vi "Array to File.vi"(8 "error in":errorcluster, 10 "array in":T1[](array[typedef]) {"Creation Date" format="%<%x>T"; "Last Updated" format="%<%x>T"}, 11 "file path in":path) -> (0 "error out":errorcluster, 3 "file path out":path)   [LabVIEW 2018]
uses:
  Type Defs/SR Cluster.ctl
  Type Defs/SR Status.ctl
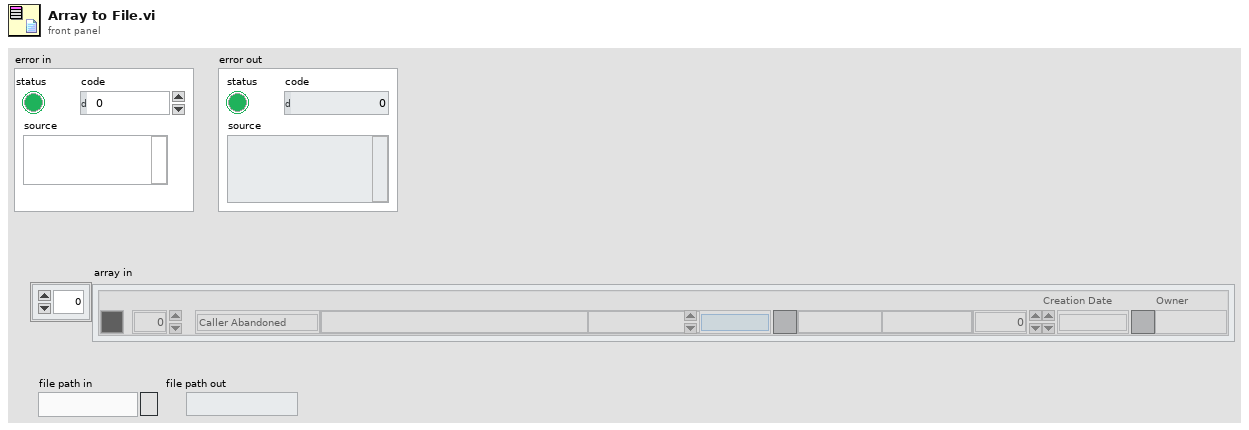
[diagram p1: front panel]
types:
  T1 = typedef "SR Cluster.ctl" = cluster{"Color":u32, "SR Number":i32, "SR Status":T2, "Name":string, "Summary":string, "Last Updated":timestamp, "SR Type":string, "Service Level":string, "Days Open":dbl, "Creation Date":timestamp, "Owner":string}
  T2 = typedef "SR Status.ctl" = enum16{"Caller Abandoned", "Created in Error", "Expired", "Forum Resolved AE", "Forum Resolved Customer", "IN WORK", "IN WORK Collab with AES", "IN WORK Collab with PSE", "IN WORK Collab with SE", "IN WORK Customer Added Note", "IN WORK Escalation", "IN WORK Wait on Customer", "Open", "Potentially Resolved", "Presumed Resolved", "RMA Approved for Return", "RMA Closed", "RMA Closed - DOA", "RMA In Progress", "RMA Open", "RMA Waiting on Customer", "Resolved", "Passed Off"}
  T3 = enum16{"open", "replace", "create", "open or create", "replace or create", "replace or create with confirmation"}
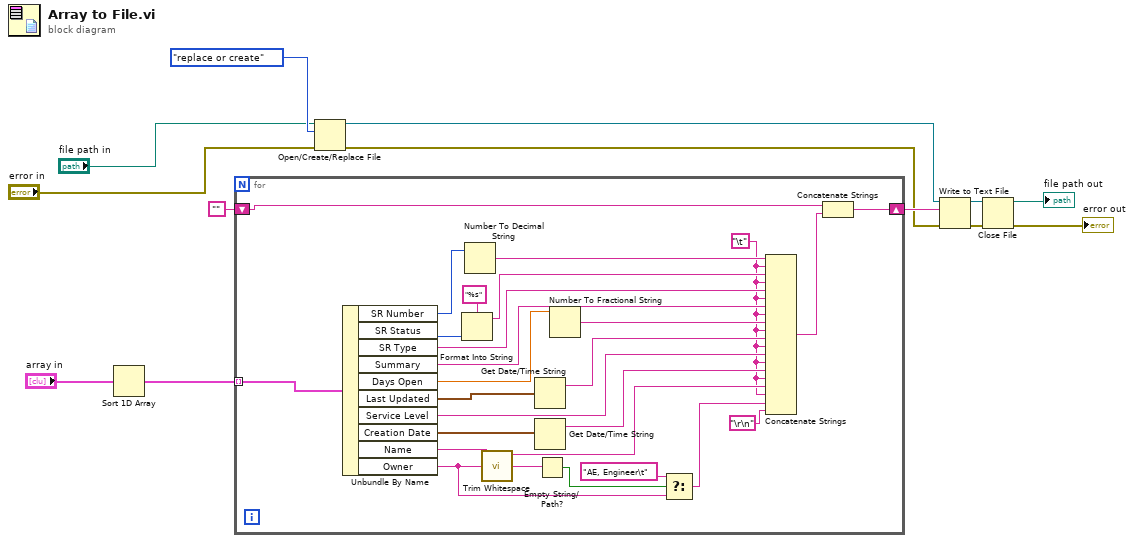
[diagram p0: block diagram]
diagram:
  n1 = Sort 1D Array(array="array in") -> (sorted array=w1:T1[])
  n2 = for {
    shift-right: [w39] -> w11
    shift-left: "" -> [w38]
    tunnel: w1 -> [w24] mode=indexing
    w15 = "\t"
    n3 = Unbundle By Name(w24) -> ("SR Number"=w36:i32, "SR Status"=w27:T2, "SR Type"=w34:string, "Summary"=w28:string, "Days Open"=w33:dbl, "Last Updated"=w29:timestamp, "Service Level"=w30:string, "Creation Date"=w23:timestamp, "Name"=w21:string, "Owner"=w17:string)
    n4 = Format Into String(format string="%s", w27) -> (resulting string=w25:string)  [unwired: 2 in, 1 out]
    n5 = Number To Decimal String(number=w36) -> (decimal integer string=w35:string)  [unwired: 1 in]
    n6 = call <vilib>:"Trim Whitespace.vi"("string"=w17) -> ("trimmed string"=w19:string)  [unwired: 1 in]
    n7 = Get Date/Time String(seconds (now)=w29) -> (date string=w31:string)  [unwired: 2 in, 1 out]
    n8 = Get Date/Time String(seconds (now)=w23) -> (date string=w22:string)  [unwired: 2 in, 1 out]
    n9 = Empty String/Path?(string/path=w19) -> (empty?=w18:bool)
    n10 = Number To Fractional String(number=w33) -> (F-format string=w32:string)  [unwired: 3 in]
    n11 = Select(t="AE, Engineer\t", s=w18, f=w17) -> (s? t:f=w14:string)
    n12 = Concatenate Strings(w35, w15, w25, w15, w34, w15, w28, w15, w32, w15, w31, w15, w30, w15, w22, w15, w21, w15, w14, "\r\n") -> (w37:string)
    n13 = Concatenate Strings(w38, w37) -> (w39:string)
  }
  n14 = Open/Create/Replace File(file path (use dialog)="file path in", error in="error in", operation (0:open)=T3."replace or create") -> (refnum out=w9:refnum<file>, error out=w10:errorcluster)  [unwired: 3 in, 1 out]
  n15 = Write to Text File(file (use dialog)=w9, text=w11, error in=w10) -> (refnum out=w7:refnum<file>, error out=w8:errorcluster)  [unwired: 1 in, 1 out]
  n16 = Close File(refnum=w7, error in=w8) -> (path=→"file path out":path, error out=→"error out":errorcluster)
